vi "Test Cases - Datatype Check.vi"() -> ()   [LabVIEW 2017]
uses:
  API-String-Arugments-Support/API String Arguments Support.lvlib
panel:
  out "String 24":string="abcd"
  out "String 23":string="Enable"
  out "String 22":string="0x42"
  out "String 21":string="3.1415926"
  out "String 20":string="bbbb"
  out "String 19":string="555"
  out "String 18":string="ccccc"
  out "String 17":string="[3.12,4.11,5]"
  out "String 16":string="Bool:Off;child.name:ddd"
  out "String 15":string="C:\\ni-rt\\data\\a\\2023.07.25"
  out "String 14":string="[{Bool:Off;child.name:ddd},{Bool:On;name:ddd}]"
  out "String 13":string="[3.12,4.113,2.3,5;3.12,5,2.3;3.12,4.11,5]"
  in  "String 12":string="[3.12,4.113,2.3,5;3.12,5,2.3;3.12,4.11,5]"
  out "error 12":errorcluster
  out "Data 11":dbl[][](array[numeric])=[[3.12, 4.113, 2.3, 5.0, 5.0, 2.3, 4.11, 5.0]]
  in  "String 11":string="[{Bool:Off;child.name:ddd},{Bool:On;name:ddd}]"
  out "error 11":errorcluster
  out "Data 10":T1(array[cluster])=[{"Name"="", "Child"={"Name"="ddd"}, "Bool"=FALSE}, {"Name"="ddd", "Child"={"Name"=""}, "Bool"=TRUE}]
  in  "String 10":string="C:\\ni-rt\\data\\a\\2023.07.25"
  out "error 10":errorcluster
  out "Data 9":path=path "C:/ni-rt/data/a/2023.07.25"
  in  "String 9":string="Bool:Off;child.name:ddd"
  out "error 9":errorcluster
  out "Data 8":T2={"Name"="abc", "Child"={"Name"="ddd"}, "Bool"=FALSE}
  in  "String 8":string="[3.12,4.11,5]"
  out "error 8":errorcluster
  out "Data 4":dbl[](array[numeric])=[3.12, 4.11, 5.0]
  in  "String 7":string="ccccc"
  out "error 7":errorcluster
  out "Data 7":enum16{"1 - aaaa", "2 - bbbb", "555 - ccccc"}(ring)=enum."555 - ccccc"
  in  "String 6":string="555"
  out "error 6":errorcluster
  out "Data 6":enum16{"1 - aaaa", "2 - bbbb", "555 - ccccc"}(ring)=enum."555 - ccccc"
  in  "String 5":string="bbbb"
  out "error 5":errorcluster
  out "Data 5":enum16{"aaaa", "bbbb", "ccccc"}(ring)=enum."bbbb"
  in  "String 4":string="3.1415926"
  out "error 4":errorcluster
  out "Data 4":dbl=3.1415926
  in  "String 3":string="0x42"
  out "error 3":errorcluster
  out "Data 3":i32=66
  in  "String 2":string="Enable"
  out "error 2":errorcluster
  out "Data 2":bool=TRUE
  out "Data 1":string="abcd"
  out "error 1":errorcluster
  in  "String":string="abcd"
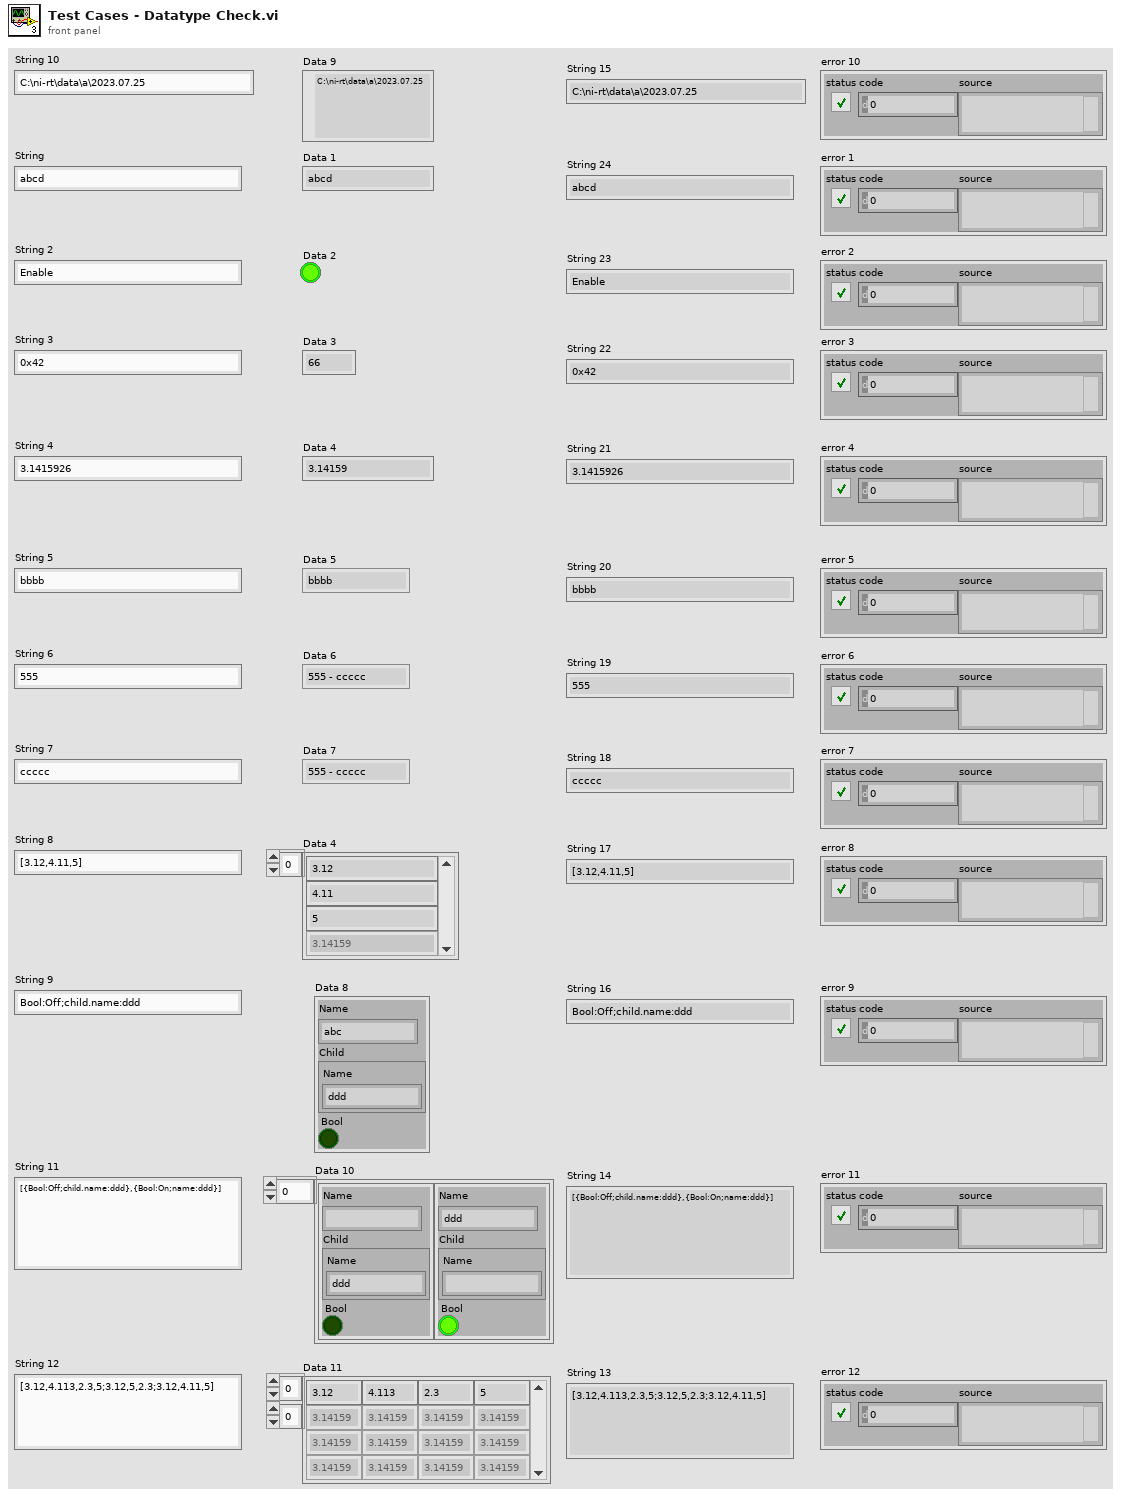
[diagram p1: front panel]
types:
  T1 = cluster{"Name":string, "Child":cluster{"Name":string}, "Bool":bool}[]
  T2 = cluster{"Name":string, "Child":cluster{"Name":string}, "Bool":bool}
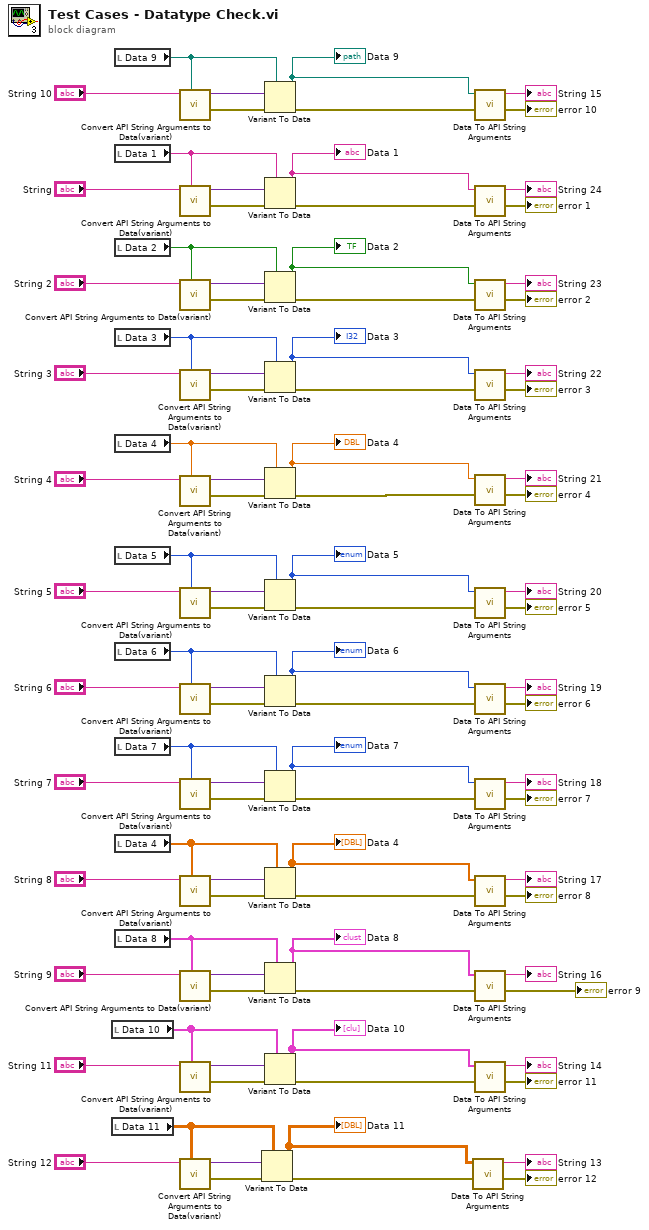
[diagram p0: block diagram]
diagram:
  n1 = local read "Data 10"() -> (w53:T1)
  n2 = local read "Data 11"() -> (w49:dbl[][])
  n3 = local read "Data 9"() -> (w57:path)
  n4 = local read "Data 1"() -> (w96:string)
  n5 = local read "Data 2"() -> (w95:bool)
  n6 = local read "Data 3"() -> (w94:i32)
  n7 = local read "Data 4"() -> (w93:dbl)
  n8 = local read "Data 5"() -> (w92:enum16{"aaaa", "bbbb", "ccccc"})
  n9 = local read "Data 6"() -> (w91:enum16{"1 - aaaa", "2 - bbbb", "555 - ccccc"})
  n10 = local read "Data 7"() -> (w90:enum16{"1 - aaaa", "2 - bbbb", "555 - ccccc"})
  n11 = local read "Data 4"() -> (w89:dbl[])
  n12 = local read "Data 8"() -> (w88:T2)
  n13 = call "Convert API String Arguments to Data(variant).vi"("Type"=w57, "String"="String 10") -> ("error"=w59:errorcluster, "Data"=w58:variant)  [unwired: 8 in]
  n14 = call "Convert API String Arguments to Data(variant).vi"("Type"=w96, "String"="String") -> ("error"=w62:errorcluster, "Data"=w63:variant)  [unwired: 8 in]
  n15 = call "Convert API String Arguments to Data(variant).vi"("Type"=w95, "String"="String 2") -> ("error"=w86:errorcluster, "Data"=w85:variant)  [unwired: 8 in]
  n16 = call "Convert API String Arguments to Data(variant).vi"("Type"=w94, "String"="String 3") -> ("error"=w83:errorcluster, "Data"=w84:variant)  [unwired: 8 in]
  n17 = call "Convert API String Arguments to Data(variant).vi"("Type"=w93, "String"="String 4") -> ("error"=w81:errorcluster, "Data"=w82:variant)  [unwired: 8 in]
  n18 = call "Convert API String Arguments to Data(variant).vi"("Type"=w92, "String"="String 5") -> ("error"=w79:errorcluster, "Data"=w80:variant)  [unwired: 8 in]
  n19 = call "Convert API String Arguments to Data(variant).vi"("Type"=w91, "String"="String 6") -> ("error"=w77:errorcluster, "Data"=w78:variant)  [unwired: 8 in]
  n20 = call "Convert API String Arguments to Data(variant).vi"("Type"=w90, "String"="String 7") -> ("error"=w75:errorcluster, "Data"=w76:variant)  [unwired: 8 in]
  n21 = call "Convert API String Arguments to Data(variant).vi"("Type"=w89, "String"="String 8") -> ("error"=w73:errorcluster, "Data"=w74:variant)  [unwired: 8 in]
  n22 = call "Convert API String Arguments to Data(variant).vi"("Type"=w88, "String"="String 9") -> ("error"=w71:errorcluster, "Data"=w72:variant)  [unwired: 8 in]
  n23 = call "Convert API String Arguments to Data(variant).vi"("Type"=w53, "String"="String 11") -> ("error"=w55:errorcluster, "Data"=w54:variant)  [unwired: 8 in]
  n24 = call "Convert API String Arguments to Data(variant).vi"("Type"=w49, "String"="String 12") -> ("error"=w51:errorcluster, "Data"=w50:variant)  [unwired: 8 in]
  n25 = Variant To Data(error in=w51, type=w49, Variant=w50) -> (data=w9:dbl[][], error out=w13:errorcluster)
  "Data 11" <- w9
  n26 = Variant To Data(error in=w59, type=w57, Variant=w58) -> (data=w1:path, error out=w24:errorcluster)
  "Data 9" <- w1
  n27 = Variant To Data(error in=w62, type=w96, Variant=w63) -> (data=w2:string, error out=w23:errorcluster)
  "Data 1" <- w2
  n28 = Variant To Data(error in=w86, type=w95, Variant=w85) -> (data=w3:bool, error out=w22:errorcluster)
  "Data 2" <- w3
  n29 = Variant To Data(error in=w83, type=w94, Variant=w84) -> (data=w4:i32, error out=w21:errorcluster)
  "Data 3" <- w4
  n30 = Variant To Data(error in=w81, type=w93, Variant=w82) -> (data=w5:dbl, error out=w20:errorcluster)
  "Data 4" <- w5
  n31 = Variant To Data(error in=w79, type=w92, Variant=w80) -> (data=w8:enum16{"aaaa", "bbbb", "ccccc"}, error out=w19:errorcluster)
  "Data 5" <- w8
  n32 = Variant To Data(error in=w77, type=w91, Variant=w78) -> (data=w7:enum16{"1 - aaaa", "2 - bbbb", "555 - ccccc"}, error out=w18:errorcluster)
  "Data 6" <- w7
  n33 = Variant To Data(error in=w75, type=w90, Variant=w76) -> (data=w6:enum16{"1 - aaaa", "2 - bbbb", "555 - ccccc"}, error out=w17:errorcluster)
  "Data 7" <- w6
  n34 = Variant To Data(error in=w73, type=w89, Variant=w74) -> (data=w12:dbl[], error out=w16:errorcluster)
  "Data 4" <- w12
  n35 = Variant To Data(error in=w71, type=w88, Variant=w72) -> (data=w11:T2, error out=w15:errorcluster)
  "Data 8" <- w11
  n36 = Variant To Data(error in=w55, type=w53, Variant=w54) -> (data=w10:T1, error out=w14:errorcluster)
  "Data 10" <- w10
  n37 = call "Data To API String Arguments.vi"("error in (no error)"=w13, "data"=w9) -> ("error out"=→"error 12":errorcluster, "String"=→"String 13":string)  [unwired: 8 in]
  n38 = call "Data To API String Arguments.vi"("error in (no error)"=w24, "data"=w1) -> ("error out"=→"error 10":errorcluster, "String"=→"String 15":string)  [unwired: 8 in]
  n39 = call "Data To API String Arguments.vi"("error in (no error)"=w23, "data"=w2) -> ("error out"=→"error 1":errorcluster, "String"=→"String 24":string)  [unwired: 8 in]
  n40 = call "Data To API String Arguments.vi"("error in (no error)"=w22, "data"=w3) -> ("error out"=→"error 2":errorcluster, "String"=→"String 23":string)  [unwired: 8 in]
  n41 = call "Data To API String Arguments.vi"("error in (no error)"=w21, "data"=w4) -> ("error out"=→"error 3":errorcluster, "String"=→"String 22":string)  [unwired: 8 in]
  n42 = call "Data To API String Arguments.vi"("error in (no error)"=w20, "data"=w5) -> ("error out"=→"error 4":errorcluster, "String"=→"String 21":string)  [unwired: 8 in]
  n43 = call "Data To API String Arguments.vi"("error in (no error)"=w19, "data"=w8) -> ("error out"=→"error 5":errorcluster, "String"=→"String 20":string)  [unwired: 8 in]
  n44 = call "Data To API String Arguments.vi"("error in (no error)"=w18, "data"=w7) -> ("error out"=→"error 6":errorcluster, "String"=→"String 19":string)  [unwired: 8 in]
  n45 = call "Data To API String Arguments.vi"("error in (no error)"=w17, "data"=w6) -> ("error out"=→"error 7":errorcluster, "String"=→"String 18":string)  [unwired: 8 in]
  n46 = call "Data To API String Arguments.vi"("error in (no error)"=w16, "data"=w12) -> ("error out"=→"error 8":errorcluster, "String"=→"String 17":string)  [unwired: 8 in]
  n47 = call "Data To API String Arguments.vi"("error in (no error)"=w15, "data"=w11) -> ("error out"=→"error 9":errorcluster, "String"=→"String 16":string)  [unwired: 8 in]
  n48 = call "Data To API String Arguments.vi"("error in (no error)"=w14, "data"=w10) -> ("error out"=→"error 11":errorcluster, "String"=→"String 14":string)  [unwired: 8 in]
